vi "Keithley6487_autozero.vi"(8 "error in (no error)":errorcluster, 10 "Autozero":bool, 11 "VISA resource name":refnum<visa-resource-name>) -> (0 "error out":errorcluster, 3 "VISA resource name out":refnum<visa-resource-name>)   [LabVIEW 2016]
panel:
  out "concatenated string":string
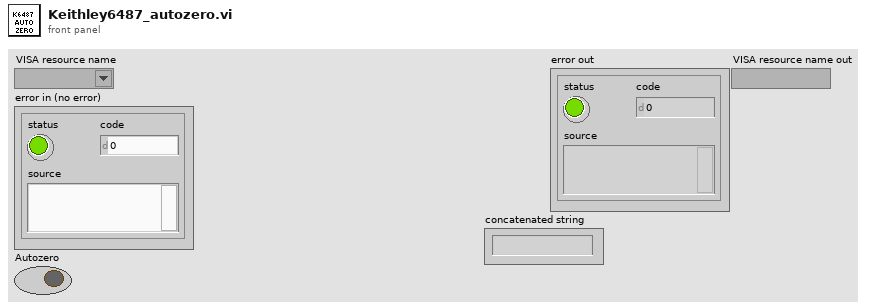
[diagram p1: front panel]
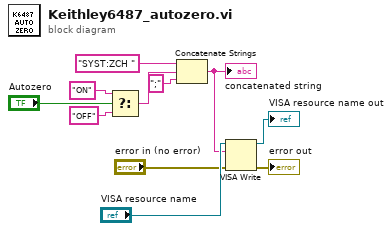
[diagram p0: block diagram]
diagram:
  n1 = Select(t="ON" ("write buffer"), s="Autozero", f="OFF" ("write buffer")) -> (s? t:f=w5:string)
  n2 = Concatenate Strings("SYST:ZCH " ("write buffer"), w5, ";" ("string")) -> (w1:string)
  "concatenated string" <- w1
  n3 = VISA Write(VISA resource name="VISA resource name", write buffer=w1, error in (no error)="error in (no error)") -> (VISA resource name out=→"VISA resource name out":refnum<visa-resource-name>, error out=→"error out":errorcluster)  [unwired: 1 out]
